vi "FaulhaberV3-Ascii_V1.vi"() -> (1 "searchnames":string[](array[string]), 2 "ID":u32[](array[numeric]), 3 "Faulhaber Objects":T3(array[cluster]))   [LabVIEW 2011] (continued)
 595132431, 595132432, 595132433, 595132434, 595132435, 595132436, 595132437, 595132438, 595132439, 595197952, 595197953, 595197954, 595197955, 595197956, 595197957, 595197958, 595197959, 595197966, 595197967, 595197968, 595197969, 595197970, 595197971, 595197972, 595197973, 595197974, 595197975, 595263488, 595263489, 595263490, 595263491, 595263492, 595263493, 595263494, 595263495, 595263502, 595263503, 595263504, 595263505, 595263506, 595263507, 595263508, 595263509, 595263510, 595263511, 595591168, 595591169, 595591170, 595591171, 595591172, 595591173, 595656704, 595656705, 595656706, 595656707, 595656708, 595656709, 595656710, 595656711, 595656712, 595722240, 595722241, 595722242, 595722243, 596574208, 596574209, 602931200, 602931201, 602931202, 602931203, 602931204, 602931205, 602931206, 602996736, 602996737, 602996738, 603127808, 603127809, 603127810, 603127811, 603127812, 603127813, 603979776, 603979777, 603979778, 603979779, 603979780, 603979781, 603979782, 603979783, 604045312, 604241920, 604307456, 604372992, 604438528, 604504064, 605028352, 605028353, 620756992, 620756993, 620756994, 620756995, 620756996, 620756997, 620756998, 620756999, 620757000, 620757001, 620757002, 620757003, 620757004, 620757005, 620757006, 620822528, 620822529, 620822530, 620822531, 620822532, 620822533, 620822534, 620822535, 620822536, 620822537, 620822538, 620822539, 620822540, 620822541, 620822542, 620888064, 620888065, 620888066, 620888067, 620888068, 620888069, 620888070, 620888071, 620888072, 620888073, 620888074, 620888075, 620888076, 620888077, 620953600, 621019136, 621019137, 621019138, 621019139, 621019140, 621019141, 621019142, 621019143, 621019144, 621019145, 621019146, 621019147, 621019148, 621150208, 621150209, 621150210, 621150211, 621150212, 621150213, 621150214, 621150215, 621150216, 621150217, 621150218, 621150219, 621150220, 621150221, 621150222, 621150223, 621150224, 621150225, 621150226, 621150227, 621150228, 621150229, 621150230, 621150231, 621150232, 621150233, 621150234, 621150235, 621150236, 621150237, 621150238, 621150239, 621150240, 621150241, 621150242, 621150243, 621150244, 621150245, 621150246, 621150247, 621150248, 621150249, 621150250, 621150251, 621150252, 621150253, 621150254, 621150255, 621150256, 621150257, 621150258, 621150259, 621150260, 621150261, 621150262, 621150263, 621150264, 621150265, 621150266, 621150267, 621150268, 621150269, 621150270, 621150271, 621150272, 621412352, 621740032, 637534208, 637534209, 637534210, 637599744, 637599745, 637599746, 637599747, 637665280, 637665281, 637665282, 637665283, 637730816, 637730817, 637730818, 637796352, 637861888, 638582784, 638582785, 638582786, 638582787, 805306368, 805306369, 805306370, 805306371, 805306372, 805306373, 805306374, 805306375, 805306376, 805371904, 805371905, 805371906, 805371907, 805371908, 805371909, 805371911, 805371912, 805371913, 805371914, 805437440, 805502976, 805568512, 805568513, 805568514, 805634048, 805634049, 805634050, 805634051, 805634052, 805634053, 805634054, 805634055, 805634056, 805634057, 805634058, 805634059, 805634060, 805634061, 805634062, 805634063, 805634064, 805634065, 805634066, 805634067, 805634068, 805634069, 805634070, 805634071, 805634072, 805634073, 805634074, 805699584, 805699585, 805699586, 805699587, 805699588, 805699589, 805699590, 805699591, 805699592, 805699593, 805699594, 805699595, 805699596, 805699597, 805699598, 805699599, 806289408, 806354944, 806354945, 806354946, 806354947, 806354948, 806354949, 806354950, 806354951, 806354952, 806354953, 806354954, 806354955, 806354956, 806354957, 806354958, 806354959, 806354960, 1611071488, 1614807040, 1614872576, 1616510976, 1616576512, 1616642048, 1616707584, 1616773120, 1616904192, 1616969728, 1617035264, 1617100800, 1617166336, 1617231872, 1617297408, 1617362944, 1617428480, 1617625088, 1617690624, 1617756160, 1617821696, 1617887232, 1617952768, 1618018304, 1618083840, 1618214912, 1618411520, 1618477056, 1618608128, 1618673664, 1618673665, 1618673666, 1618739200, 1618804736, 1618804737, 1618804738, 1618870272, 1619001344, 1619066880, 1619197952, 1619263488, 1619329024, 1619394560, 1619984384, 1619984385, 1619984386, 1620049920, 1620049921, 1620049922, 1620115456, 1620115457, 1620115458, 1620180992, 1620180993, 1620180994, 1620443136, 1620443137, 1620443138, 1620574208, 1620639744, 1620639745, 1620639746, 1620705280, 1622147072, 1622212608, 1622278144, 1622671360, 1622736896, 1622802432, 1622867968, 1622933504, 1622999040, 1623523328, 1623588864, 1624571904, 1624637440, 1624702976, 1624768512, 1625292800, 1625358336, 1626472448, 1626603520, 1627193344, 1627324416, 1677918208, 1694629888, 1694695424] format="%08x", 3 "Faulhaber Objects":T3(array[cluster])=[{"ID"=268435456, "Name"="Device type", "type"=enum."U32", "rw"=enum."ro", "lowLimit"="", "highLimit"="", "Default"="0x420192", "Kommentart"=""}, {"ID"=268500992, "Name"="Error register", "type"=enum."U8", "rw"=enum."ro", "lowLimit"="", "highLimit"="", "Default"="", "Kommentart"=""}, {"ID"=268632064, "Name"="Pre-defined error field_Number of errors", "type"=enum."U8", "rw"=enum."rw", "lowLimit"="0", "highLimit"="255", "Default"="0", "Kommentart"=""}, {"ID"=268632065, "Name"="Pre-defined error field_Standard error field 1", "type"=enum."U32", "rw"=enum."ro", "lowLimit"="", "highLimit"="", "Default"="0x0", "Kommentart"=""}, {"ID"=268632066, "Name"="Pre-defined error field_Standard error field 2", "type"=enum."U32", "rw"=enum."ro", "lowLimit"="", "highLimit"="", "Default"="0x0", "Kommentart"=""}, {"ID"=268632067, "Name"="Pre-defined error field_Standard error field 3", "type"=enum."U32", "rw"=enum."ro", "lowLimit"="", "highLimit"="", "Default"="0x0", "Kommentart"=""}, {"ID"=268632068, "Name"="Pre-defined error field_Standard error field 4", "type"=enum."U32", "rw"=enum."ro", "lowLimit"="", "highLimit"="", "Default"="0x0", "Kommentart"=""}, {"ID"=268632069, "Name"="Pre-defined error field_Standard error field 5", "type"=enum."U32", "rw"=enum."ro", "lowLimit"="", "highLimit"="", "Default"="0x0", "Kommentart"=""}, {"ID"=268632070, "Name"="Pre-defined error field_Standard error field 6", "type"=enum."U32", "rw"=enum."ro", "lowLimit"="", "highLimit"="", "Default"="0x0", "Kommentart"=""}, {"ID"=268632071, "Name"="Pre-defined error field_Standard error field 7", "type"=enum."U32", "rw"=enum."ro", "lowLimit"="", "highLimit"="", "Default"="0x0", "Kommentart"=""}, {"ID"=268632072, "Name"="Pre-defined error field_Standard error field 8", "type"=enum."U32", "rw"=enum."ro", "lowLimit"="", "highLimit"="", "Default"="0x0", "Kommentart"=""}, {"ID"=268763136, "Name"="COB-ID SYNC", "type"=enum."U32", "rw"=enum."rw", "lowLimit"="1", "highLimit"="4294967295", "Default"="0x80", "Kommentart"=""}, {"ID"=268959744, "Name"="Manufacturer device name", "type"=enum."string", "rw"=enum."const", "lowLimit"="", "highLimit"="", "Default"="", "Kommentart"=""}, {"ID"=269025280, "Name"="Manufacturer hardware version", "type"=enum."string", "rw"=enum."const", "lowLimit"="", "highLimit"="", "Default"="", "Kommentart"=""}, {"ID"=269090816, "Name"="Manufacturer software version", "type"=enum."string", "rw"=enum."const", "lowLimit"="", "highLimit"="", "Default"="", "Kommentart"=""}, {"ID"=269221888, "Name"="Guard time", "type"=enum."U16", "rw"=enum."rw", "lowLimit"="0", "highLimit"="65535", "Default"="0", "Kommentart"=""}, {"ID"=269287424, "Name"="Life time factor", "type"=enum."U8", "rw"=enum."rw", "lowLimit"="0", "highLimit"="255", "Default"="0", "Kommentart"=""}, {"ID"=269484032, "Name"="Store parameters_Number of entries", "type"=enum."U8", "rw"=enum."ro", "lowLimit"="", "highLimit"="", "Default"="9", "Kommentart"=""}, {"ID"=269484033, "Name"="Store parameters_Save all parameters", "type"=enum."U32", "rw"=enum."rw", "lowLimit"="", "highLimit"="", "Default"="", "Kommentart"=""}, {"ID"=269484034, "Name"="Store parameters_Save comm parameters", "type"=enum."U32", "rw"=enum."rw", "lowLimit"="", "highLimit"="", "Default"="", "Kommentart"=""}, {"ID"=269484035, "Name"="Store parameters_Save app parameters", "type"=enum."U32", "rw"=enum."rw", "lowLimit"="", "highLimit"="", "Default"="", "Kommentart"=""}, {"ID"=269484036, "Name"="Store parameters_Save app parameters 1", "type"=enum."U32", "rw"=enum."rw", "lowLimit"="", "highLimit"="", "Default"="", "Kommentart"=""}, {"ID"=269484037, "Name"="Store parameters_Save app parameters 2", "type"=enum."U32", "rw"=enum."rw", "lowLimit"="", "highLimit"="", "Default"="", "Kommentart"=""}, {"ID"=269484038, "Name"="Store parameters_Save cal parameters", "type"=enum."U32", "rw"=enum."ro", "lowLimit"="", "highLimit"="", "Default"="", "Kommentart"=""}, {"ID"=269484039, "Name"="Store parameters_Save factory parameter alls", "type"=enum."U32", "rw"=enum."ro", "lowLimit"="", "highLimit"="", "Default"="", "Kommentart"=""}, {"ID"=269484040, "Name"="Store parameters_Save factory parameters com", "type"=enum."U32", "rw"=enum."ro", "lowLimit"="", "highLimit"="", "Default"="", "Kommentart"=""}, {"ID"=269484041, "Name"="Store parameters_Save factory parameters app", "type"=enum."U32", "rw"=enum."ro", "lowLimit"="", "highLimit"="", "Default"="", "Kommentart"=""}, {"ID"=269549568, "Name"="Restore default parameters_Number of entries", "type"=enum."U8", "rw"=enum."ro", "lowLimit"="", "highLimit"="", "Default"="6", "Kommentart"=""}, {"ID"=269549569, "Name"="Restore default parameters_Restore all default parameters", "type"=enum."U32", "rw"=enum."rw", "lowLimit"="", "highLimit"="", "Default"="", "Kommentart"=""}, {"ID"=269549570, "Name"="Restore default parameters_Restore comm default parameters", "type"=enum."U32", "rw"=enum."rw", "lowLimit"="", "highLimit"="", "Default"="", "Kommentart"=""}, {"ID"=269549571, "Name"="Restore default parameters_Restore app default parameters", "type"=enum."U32", "rw"=enum."rw", "lowLimit"="", "highLimit"="", "Default"="", "Kommentart"=""}, {"ID"=269549572, "Name"="Restore default parameters_Restore app saved", "type"=enum."U32", "rw"=enum."rw", "lowLimit"="", "highLimit"="", "Default"="", "Kommentart"=""}, {"ID"=269549573, "Name"="Restore default parameters_Restore app 1 saved", "type"=enum."U32", "rw"=enum."rw", "lowLimit"="", "highLimit"="", "Default"="", "Kommentart"=""}, {"ID"=269549574, "Name"="Restore default parameters_Restore app 2 saved", "type"=enum."U32", "rw"=enum."rw", "lowLimit"="", "highLimit"="", "Default"="", "Kommentart"=""}, {"ID"=269746176, "Name"="COB-ID EMCY", "type"=enum."U32", "rw"=enum."rw", "lowLimit"="", "highLimit"="", "Default"="$NODEID+0x80", "Kommentart"=""}, {"ID"=269877248, "Name"="Consumer heartbeat time_Number of entries", "type"=enum."U8", "rw"=enum."ro", "lowLimit"="", "highLimit"="", "Default"="1", "Kommentart"=""}, {"ID"=269877249, "Name"="Consumer heartbeat time_Consumer heartbeat time", "type"=enum."U32", "rw"=enum."rw", "lowLimit"="0", "highLimit"="0x007FFFFF", "Default"="0x0", "Kommentart"=""}, {"ID"=269942784, "Name"="Producer heartbeat time", "type"=enum."U16", "rw"=enum."rw", "lowLimit"="0", "highLimit"="65535", "Default"="0", "Kommentart"=""}, {"ID"=270008320, "Name"="Identity object_Number of entries", "type"=enum."U8", "rw"=enum."ro", "lowLimit"="", "highLimit"="", "Default"="4", "Kommentart"=""}, {"ID"=270008321, "Name"="Identity object_Vendor ID", "type"=enum."U32", "rw"=enum."ro", "lowLimit"="", "highLimit"="", "Default"="327", "Kommentart"=""}, {"ID"=270008322, "Name"="Identity object_Product code", "type"=enum."U32", "rw"=enum."ro", "lowLimit"="", "highLimit"="", "Default"="", "Kommentart"=""}, {"ID"=270008323, "Name"="Identity object_Revision number", "type"=enum."U32", "rw"=enum."ro", "lowLimit"="0x0", "highLimit"="", "Default"="", "Kommentart"=""}, {"ID"=270008324, "Name"="Identity object_Serial number", "type"=enum."U32", "rw"=enum."ro", "lowLimit"="", "highLimit"="", "Default"="", "Kommentart"=""}, {"ID"=271122432, "Name"="Error behaviour / Number of error classes_Number of error classes", "type"=enum."U8", "rw"=enum."ro", "lowLimit"="", "highLimit"="", "Default"="1", "Kommentart"=""}, {"ID"=271122433, "Name"="Error behaviour / Number of error classes_Communication error", "type"=enum."U8", "rw"=enum."unknown", "lowLimit"="", "highLimit"="", "Default"="", "Kommentart"=""}, {"ID"=301989888, "Name"="Server SDO parameter_Number of entries", "type"=enum."U8", "rw"=enum."ro", "lowLimit"="", "highLimit"="", "Default"="2", "Kommentart"=""}, {"ID"=301989889, "Name"="Server SDO parameter_COB-ID client to server (rx)", "type"=enum."U32", "rw"=enum."ro", "lowLimit"="", "highLimit"="", "Default"="$NODEID+0x600", "Kommentart"=""}, {"ID"=301989890, "Name"="Server SDO parameter_COB-ID server to client (tx)", "type"=enum."U32", "rw"=enum."ro", "lowLimit"="", "highLimit"="", "Default"="$NODEID+0x580", "Kommentart"=""}, {"ID"=335544320, "Name"="Receive PDO1 parameter_Number of entries", "type"=enum."U8", "rw"=enum."ro", "lowLimit"="", "highLimit"="", "Default"="2", "Kommentart"=""}, {"ID"=335544321, "Name"="Receive PDO1 parameter_COB-ID used by RxPDO1", "type"=enum."U32", "rw"=enum."rw", "lowLimit"="1", "highLimit"="4294967295", "Default"="$NODEID+0x200", "Kommentart"=""}, {"ID"=335544322, "Name"="Receive PDO1 parameter_Transmission type", "type"=enum."U8", "rw"=enum."rw", "lowLimit"="0", "highLimit"="255", "Default"="255", "Kommentart"=""}, {"ID"=335609856, "Name"="Receive PDO2 parameter_Number of entries", "type"=enum."U8", "rw"=enum."ro", "lowLimit"="", "highLimit"="", "Default"="2", "Kommentart"=""}, {"ID"=335609857, "Name"="Receive PDO2 parameter_COB-ID used by RxPDO2", "type"=enum."U32", "rw"=enum."rw", "lowLimit"="1", "highLimit"="4294967295", "Default"="$NODEID+0x300", "Kommentart"=""}, {"ID"=335609858, "Name"="Receive PDO2 parameter_Transmission type", "type"=enum."U8", "rw"=enum."rw", "lowLimit"="0", "highLimit"="255", "Default"="255", "Kommentart"=""}, {"ID"=335675392, "Name"="Receive PDO3 parameters_Number of entries", "type"=enum."U8", "rw"=enum."ro", "lowLimit"="", "highLimit"="", "Default"="2", "Kommentart"=""}, {"ID"=335675393, "Name"="Receive PDO3 parameters_COB-ID used by RxPDO3", "type"=enum."U32", "rw"=enum."rw", "lowLimit"="1", "highLimit"="4294967295", "Default"="$NODEID+0x400", "Kommentart"=""}, {"ID"=335675394, "Name"="Receive PDO3 parameters_Transmission type", "type"=enum."U8", "rw"=enum."rw", "lowLimit"="0", "highLimit"="255", "Default"="255", "Kommentart"=""}, {"ID"=335740928, "Name"="Receive PDO4 parameter_Number of entries", "type"=enum."U8", "rw"=enum."ro", "lowLimit"="", "highLimit"="", "Default"="2", "Kommentart"=""}, {"ID"=335740929, "Name"="Receive PDO4 parameter_COB-ID used by RxPDO4", "type"=enum."U32", "rw"=enum."rw", "lowLimit"="1", "highLimit"="4294967295", "Default"="$NODEID+0x500", "Kommentart"=""}, {"ID"=335740930, "Name"="Receive PDO4 parameter_Transmission type", "type"=enum."U8", "rw"=enum."rw", "lowLimit"="0", "highLimit"="255", "Default"="255", "Kommentart"=""}, {"ID"=369098752, "Name"="Receive PDO1 mapping / Number of mapped objects_Number of mapped objects", "type"=enum."U8", "rw"=enum."rw", "lowLimit"="0", "highLimit"="4", "Default"="1", "Kommentart"=""}, {"ID"=369098753, "Name"="Receive PDO1 mapping / Number of mapped objects_RxPDO 1 mapping entry 1", "type"=enum."U32", "rw"=enum."rw", "lowLimit"="0", "highLimit"="4294967295", "Default"="0x60400010", "Kommentart"=""}, {"ID"=369098754, "Name"="Receive PDO1 mapping / Number of mapped objects_RxPDO 1 Mapping entry 2", "type"=enum."U32", "rw"=enum."rw", "lowLimit"="0", "highLimit"="4294967295", "Default"="0x0", "Kommentart"=""}, {"ID"=369098755, "Name"="Receive PDO1 mapping / Number of mapped objects_RxPDO 1 Mapping entry 3", "type"=enum."U32", "rw"=enum."rw", "lowLimit"="0", "highLimit"="4294967295", "Default"="0x0", "Kommentart"=""}, {"ID"=369098756, "Name"="Receive PDO1 mapping / Number of mapped objects_RxPDO 1 Mapping entry 4", "type"=enum."U32", "rw"=enum."rw", "lowLimit"="0", "highLimit"="4294967295", "Default"="0x0", "Kommentart"=""}, {"ID"=369164288, "Name"="Receive PDO2 mapping / Number of mapped objects_Number of mapped objects", "type"=enum."U8", "rw"=enum."rw", "lowLimit"="0", "highLimit"="4", "Default"="2", "Kommentart"=""}, {"ID"=369164289, "Name"="Receive PDO2 mapping / Number of mapped objects_RxPDO2 mapping entry 1", "type"=enum."U32", "rw"=enum."rw", "lowLimit"="0", "highLimit"="4294967295", "Default"="0x60400010", "Kommentart"=""}, {"ID"=369164290, "Name"="Receive PDO2 mapping / Number of mapped objects_RxPDO2 mapping entry 2", "type"=enum."U32", "rw"=enum."rw", "lowLimit"="0", "highLimit"="4294967295", "Default"="0x607A0020", "Kommentart"=""}, {"ID"=369164291, "Name"="Receive PDO2 mapping / Number of mapped objects_RxPDO2 mapping entry 3", "type"=enum."U32", "rw"=enum."rw", "lowLimit"="0", "highLimit"="4294967295", "Default"="0x0", "Kommentart"=""}, {"ID"=369164292, "Name"="Receive PDO2 mapping / Number of mapped objects_RxPDO2 mapping entry 4", "type"=enum."U32", "rw"=enum."rw", "lowLimit"="0", "highLimit"="4294967295", "Default"="0x0", "Kommentart"=""}, {"ID"=369229824, "Name"="Receive PDO3 mapping / Number of mapped objects_Number of mapped objects", "type"=enum."U8", "rw"=enum."rw", "lowLimit"="0", "highLimit"="4", "Default"="2", "Kommentart"=""}, {"ID"=369229825, "Name"="Receive PDO3 mapping / Number of mapped objects_RxPDO3 mapping entry 1", "type"=enum."U32", "rw"=enum."rw", "lowLimit"="0", "highLimit"="4294967295", "Default"="0x60400010", "Kommentart"=""}, {"ID"=369229826, "Name"="Receive PDO3 mapping / Number of mapped objects_RxPDO3 mapping entry 2", "type"=enum."U32", "rw"=enum."rw", "lowLimit"="0", "highLimit"="4294967295", "Default"="0x60FF0020", "Kommentart"=""}, {"ID"=369229827, "Name"="Receive PDO3 mapping / Number of mapped objects_RxPDO3 mapping entry 3", "type"=enum."U32", "rw"=enum."rw", "lowLimit"="0", "highLimit"="4294967295", "Default"="0x0", "Kommentart"=""}, {"ID"=369229828, "Name"="Receive PDO3 mapping / Number of mapped objects_RxPDO3 mapping entry 4", "type"=enum."U32", "rw"=enum."rw", "lowLimit"="0", "highLimit"="4294967295", "Default"="0x0", "Kommentart"=""}, {"ID"=369295360, "Name"="Receive PDO4 mapping / Number of mapped objects_Number of mapped objects", "type"=enum."U8", "rw"=enum."rw", "lowLimit"="0", "highLimit"="4", "Default"="2", "Kommentart"=""}, {"ID"=369295361, "Name"="Receive PDO4 mapping / Number of mapped objects_RxPDO4 mapping entry 1", "type"=enum."U32", "rw"=enum."rw", "lowLimit"="0", "highLimit"="4294967295", "Default"="0x60400010", "Kommentart"=""}, {"ID"=369295362, "Name"="Receive PDO4 mapping / Number of mapped objects_RxPDO4 mapping entry 2", "type"=enum."U32", "rw"=enum."rw", "lowLimit"="0", "highLimit"="4294967295", "Default"="0x60710010", "Kommentart"=""}, {"ID"=369295363, "Name"="Receive PDO4 mapping / Number of mapped objects_RxPDO4 mapping entry 3", "type"=enum."U32", "rw"=enum."rw", "lowLimit"="0", "highLimit"="4294967295", "Default"="0x0", "Kommentart"=""}, {"ID"=369295364, "Name"="Receive PDO4 mapping / Number of mapped objects_RxPDO4 mapping entry 4", "type"=enum."U32", "rw"=enum."rw", "lowLimit"="0", "highLimit"="4294967295", "Default"="0x0", "Kommentart"=""}, {"ID"=402653184, "Name"="Transmit PDO1 parameter_Number of entries", "type"=enum."U8", "rw"=enum."ro", "lowLimit"="", "highLimit"="", "Default"="5", "Kommentart"=""}, {"ID"=402653185, "Name"="Transmit PDO1 parameter_COB-ID used by TxPDO1", "type"=enum."U32", "rw"=enum."rw", "lowLimit"="1", "highLimit"="4294967295", "Default"="$NODEID+0x180", "Kommentart"=""}, {"ID"=402653186, "Name"="Transmit PDO1 parameter_Transmission type", "type"=enum."U8", "rw"=enum."rw", "lowLimit"="0", "highLimit"="255", "Default"="255", "Kommentart"=""}, {"ID"=402653189, "Name"="Transmit PDO1 parameter_Eventtimer", "type"=enum."U16", "rw"=enum."rw", "lowLimit"="0", "highLimit"="65535", "Default"="0", "Kommentart"=""}, {"ID"=402718720, "Name"="Transmit PDO2 parameter_Number of entries", "type"=enum."U8", "rw"=enum."ro", "lowLimit"="", "highLimit"="", "Default"="5", "Kommentart"=""}, {"ID"=402718721, "Name"="Transmit PDO2 parameter_COB-ID used by TxPDO2", "type"=enum."U32", "rw"=enum."rw", "lowLimit"="1", "highLimit"="4294967295", "Default"="$NODEID+0x280", "Kommentart"=""}, {"ID"=402718722, "Name"="Transmit PDO2 parameter_Transmission type", "type"=enum."U8", "rw"=enum."rw", "lowLimit"="0", "highLimit"="255", "Default"="255", "Kommentart"=""}, {"ID"=402718725, "Name"="Transmit PDO2 parameter_Eventtimer", "type"=enum."U16", "rw"=enum."rw", "lowLimit"="0", "highLimit"="65535", "Default"="0", "Kommentart"=""}, {"ID"=402784256, "Name"="Transmit PDO3 parameter_Number of entries", "type"=enum."U8", "rw"=enum."ro", "lowLimit"="", "highLimit"="", "Default"="5", "Kommentart"=""}, {"ID"=402784257, "Name"="Transmit PDO3 parameter_COB-ID used by TxPDO3", "type"=enum."U32", "rw"=enum."rw", "lowLimit"="1", "highLimit"="4294967295", "Default"="$NODEID+0x380", "Kommentart"=""}, {"ID"=402784258, "Name"="Transmit PDO3 parameter_Transmission type", "type"=enum."U8", "rw"=enum."rw", "lowLimit"="0", "highLimit"="255", "Default"="255", "Kommentart"=""}, {"ID"=402784261, "Name"="Transmit PDO3 parameter_Eventtimer", "type"=enum."U16", "rw"=enum."rw", "lowLimit"="0", "highLimit"="65535", "Default"="0", "Kommentart"=""}, {"ID"=402849792, "Name"="Transmit PDO4 parameter_Number of entries", "type"=enum."U8", "rw"=enum."ro", "lowLimit"="", "highLimit"="", "Default"="5", "Kommentart"=""}, {"ID"=402849793, "Name"="Transmit PDO4 parameter_COB-ID used by TxPDO4", "type"=enum."U32", "rw"=enum."rw", "lowLimit"="1", "highLimit"="4294967295", "Default"="$NODEID+0x480", "Kommentart"=""}, {"ID"=402849794, "Name"="Transmit PDO4 parameter_Transmission type", "type"=enum."U8", "rw"=enum."rw", "lowLimit"="0", "highLimit"="255", "Default"="255", "Kommentart"=""}, {"ID"=402849797, "Name"="Transmit PDO4 parameter_Eventtimer", "type"=enum."U16", "rw"=enum."rw", "lowLimit"="0", "highLimit"="65535", "Default"="0", "Kommentart"=""}, {"ID"=436207616, "Name"="Transmit PDO1 mapping  / Number of mapped objects_Number of mapped objects", "type"=enum."U8", "rw"=enum."rw", "lowLimit"="0", "highLimit"="4", "Default"="1", "Kommentart"=""}, {"ID"=436207617, "Name"="Transmit PDO1 mapping  / Number of mapped objects_TPDO1 mapping entry 1", "type"=enum."U32", "rw"=enum."rw", "lowLimit"="0", "highLimit"="4294967295", "Default"="0x60410010", "Kommentart"=""}, {"ID"=436207618, "Name"="Transmit PDO1 mapping  / Number of mapped objects_TPDO1 mapping entry 2", "type"=enum."U32", "rw"=enum."rw", "lowLimit"="0", "highLimit"="4294967295", "Default"="0x0", "Kommentart"=""}, {"ID"=436207619, "Name"="Transmit PDO1 mapping  / Number of mapped objects_TxPDO1 mapping entry 3", "type"=enum."U32", "rw"=enum."rw", "lowLimit"="0", "highLimit"="4294967295", "Default"="0x0", "Kommentart"=""}, {"ID"=436207620, "Name"="Transmit PDO1 mapping  / Number of mapped objects_TxPDO1 mapping entry 4", "type"=enum."U32", "rw"=enum."rw", "lowLimit"="0", "highLimit"="4294967295", "Default"="0x0", "Kommentart"=""}, {"ID"=436273152, "Name"="Transmit PDO2 mapping  / Number of mapped objects_Number of mapped objects", "type"=enum."U8", "rw"=enum."rw", "lowLimit"="0", "highLimit"="4", "Default"="2", "Kommentart"=""}, {"ID"=436273153, "Name"="Transmit PDO2 mapping  / Number of mapped objects_TxPDO1 mapping entry 1", "type"=enum."U32", "rw"=enum."rw", "lowLimit"="0", "highLimit"="4294967295", "Default"="0x60410010", "Kommentart"=""}, {"ID"=436273154, "Name"="Transmit PDO2 mapping  / Number of mapped objects_TxPDO2 mapping entry 2", "type"=enum."U32", "rw"=enum."rw", "lowLimit"="0", "highLimit"="4294967295", "Default"="0x60640020", "Kommentart"=""}, {"ID"=436273155, "Name"="Transmit PDO2 mapping  / Number of mapped objects_TxPDO3 mapping entry 3", "type"=enum."U32", "rw"=enum."rw", "lowLimit"="0", "highLimit"="4294967295", "Default"="0x0", "Kommentart"=""}, {"ID"=436273156, "Name"="Transmit PDO2 mapping  / Number of mapped objects_TxPDO4 mapping entry 4", "type"=enum."U32", "rw"=enum."rw", "lowLimit"="0", "highLimit"="4294967295", "Default"="0x0", "Kommentart"=""}, {"ID"=436338688, "Name"="Transmit PDO3 mapping  / Number of mapped objects_Number of mapped objects", "type"=enum."U8", "rw"=enum."rw", "lowLimit"="0", "highLimit"="4", "Default"="2", "Kommentart"=""}, {"ID"=436338689, "Name"="Transmit PDO3 mapping  / Number of mapped objects_TxPDO3 mapping entry 1", "type"=enum."U32", "rw"=enum."rw", "lowLimit"="0", "highLimit"="4294967295", "Default"="0x60410010", "Kommentart"=""}, {"ID"=436338690, "Name"="Transmit PDO3 mapping  / Number of mapped objects_TxPDO3 mapping entry 2", "type"=enum."U32", "rw"=enum."rw", "lowLimit"="0", "highLimit"="4294967295", "Default"="0x606C0020", "Kommentart"=""}, {"ID"=436338691, "Name"="Transmit PDO3 mapping  / Number of mapped objects_TxPDO3 mapping entry 3", "type"=enum."U32", "rw"=enum."rw", "lowLimit"="0", "highLimit"="4294967295", "Default"="0x0", "Kommentart"=""}, {"ID"=436338692, "Name"="Transmit PDO3 mapping  / Number of mapped objects_TxPDO3 mapping entry 4", "type"=enum."U32", "rw"=enum."rw", "lowLimit"="0", "highLimit"="4294967295", "Default"="0x0", "Kommentart"=""}, {"ID"=436404224, "Name"="Transmit PDO4 mapping  / Number of mapped objects_Number of mapped objects", "type"=enum."U8", "rw"=enum."rw", "lowLimit"="0", "highLimit"="4", "Default"="2", "Kommentart"=""}, {"ID"=436404225, "Name"="Transmit PDO4 mapping  / Number of mapped objects_TxPDO4 mapping entry 1", "type"=enum."U32", "rw"=enum."rw", "lowLimit"="0", "highLimit"="4294967295", "Default"="0x60410010", "Kommentart"=""}, {"ID"=436404226, "Name"="Transmit PDO4 mapping  / Number of mapped objects_TxPDO4 mapping entry 2", "type"=enum."U32", "rw"=enum."rw", "lowLimit"="0", "highLimit"="4294967295", "Default"="0x60770010", "Kommentart"=""}, {"ID"=436404227, "Name"="Transmit PDO4 mapping  / Number of mapped objects_TxPDO4 mapping entry 3", "type"=enum."U32", "rw"=enum."rw", "lowLimit"="0", "highLimit"="4294967295", "Default"="0x0", "Kommentart"=""}, {"ID"=436404228, "Name"="Transmit PDO4 mapping  / Number of mapped objects_TxPDO4 mapping entry 4", "type"=enum."U32", "rw"=enum."rw", "lowLimit"="0", "highLimit"="4294967295", "Default"="0x0", "Kommentart"=""}, {"ID"=587202560, "Name"="Number of I/Os_Number of entries", "type"=enum."U8", "rw"=enum."ro", "lowLimit"="", "highLimit"="", "Default"="4", "Kommentart"=""}, {"ID"=587202561, "Name"="Number of I/Os_Number of digital inputs", "type"=enum."U8", "rw"=enum."ro", "lowLimit"="", "highLimit"="", "Default"="", "Kommentart"=""}, {"ID"=587202562, "Name"="Number of I/Os_Number of digital outputs", "type"=enum."U8", "rw"=enum."ro", "lowLimit"="", "highLimit"="", "Default"="", "Kommentart"=""}, {"ID"=587202563, "Name"="Number of I/Os_Number of analog inputs", "type"=enum."U8", "rw"=enum."ro", "lowLimit"="", "highLimit"="", "Default"="", "Kommentart"=""}, {"ID"=587202564, "Name"="Number of I/Os_Number of emulated digital inputs", "type"=enum."U8", "rw"=enum."unknown", "lowLimit"="", "highLimit"="", "Default"="", "Kommentart"=""}, {"ID"=588251136, "Name"="Digital input settings_Number of entries", "type"=enum."U8", "rw"=enum."ro", "lowLimit"="", "highLimit"="", "Default"="18", "Kommentart"=""}, {"ID"=588251137, "Name"="Digital input settings_Select lower limit switch inputs", "type"=enum."U8", "rw"=enum."unknown", "lowLimit"="", "highLimit"="", "Default"="", "Kommentart"=""}, {"ID"=588251138, "Name"="Digital input settings_Select upper limit switch inputs", "type"=enum."U8", "rw"=enum."unknown", "lowLimit"="", "highLimit"="", "Default"="", "Kommentart"=""}, {"ID"=588251139, "Name"="Digital input settings_Limit switch option code", "type"=enum."S16", "rw"=enum."unknown", "lowLimit"="", "highLimit"="", "Default"="", "Kommentart"=""}, {"ID"=588251140, "Name"="Digital input settings_Select reference switch input", "type"=enum."U8", "rw"=enum."rw", "lowLimit"="0", "highLimit"="8", "Default"="0", "Kommentart"=""}, {"ID"=588251141, "Name"="Digital input settings_Emulated input threshold level", "type"=enum."U8", "rw"=enum."rw", "lowLimit"="0", "highLimit"="0x03", "Default"="0x00", "Kommentart"=""}, {"ID"=588251142, "Name"="Digital input settings_Select stop input", "type"=enum."U8", "rw"=enum."unknown", "lowLimit"="", "highLimit"="", "Default"="", "Kommentart"=""}, {"ID"=588251144, "Name"="Digital input settings_Debug Write Digital Input Values", "type"=enum."U8", "rw"=enum."wo", "lowLimit"="0", "highLimit"="255", "Default"="", "Kommentart"=""}, {"ID"=588251145, "Name"="Digital input settings_Debug Write Brake / Fault Pin", "type"=enum."U8", "rw"=enum."wo", "lowLimit"="0", "highLimit"="255", "Default"="", "Kommentart"=""}, {"ID"=588251151, "Name"="Digital input settings_Select digital inputs used", "type"=enum."U8", "rw"=enum."rw", "lowLimit"="0", "highLimit"="255", "Default"="0xFF", "Kommentart"=""}, {"ID"=588251152, "Name"="Digital input settings_Input polarity", "type"=enum."U8", "rw"=enum."rw", "lowLimit"="0", "highLimit"="255", "Default"="0x0", "Kommentart"=""}, {"ID"=588251153, "Name"="Digital input settings_Input threshold level", "type"=enum."U8", "rw"=enum."unknown", "lowLimit"="", "highLimit"="", "Default"="", "Kommentart"=""}, {"ID"=588251154, "Name"="Digital input settings_Input filter active", "type"=enum."U8", "rw"=enum."rw", "lowLimit"="0", "highLimit"="255", "Default"="0x0", "Kommentart"=""}, {"ID"=588316672, "Name"="Digital I/O status_Number of entries", "type"=enum."U8", "rw"=enum."ro", "lowLimit"="", "highLimit"="", "Default"="4", "Kommentart"=""}, {"ID"=588316673, "Name"="Digital I/O status_Digital input logical state", "type"=enum."U8", "rw"=enum."ro", "lowLimit"="0x0", "highLimit"="", "Default"="", "Kommentart"=""}, {"ID"=588316674, "Name"="Digital I/O status_Digital input physical state", "type"=enum."U8", "rw"=enum."ro", "lowLimit"="0x0", "highLimit"="", "Default"="", "Kommentart"=""}, {"ID"=588316675, "Name"="Digital I/O status_Digital output status", "type"=enum."U8", "rw"=enum."ro", "lowLimit"="0x0", "highLimit"="", "Default"="", "Kommentart"=""}, {"ID"=588316676, "Name"="Digital I/O status_Write digital outputs", "type"=enum."U16", "rw"=enum."rw", "lowLimit"="0", "highLimit"="65535", "Default"="0x0", "Kommentart"=""}, {"ID"=588382208, "Name"="Digital output settings_Number of entries", "type"=enum."U8", "rw"=enum."ro", "lowLimit"="", "highLimit"="", "Default"="16", "Kommentart"=""}, {"ID"=588382209, "Name"="Digital output settings_Select fault output pin", "type"=enum."U8", "rw"=enum."rw", "lowLimit"="0", "highLimit"="255", "Default"="0", "Kommentart"=""}, {"ID"=588382210, "Name"="Digital output settings_Select brake control pin", "type"=enum."U8", "rw"=enum."rw", "lowLimit"="0", "highLimit"="255", "Default"="0", "Kommentart"=""}, {"ID"=588382211, "Name"="Digital output settings_Brake delay time", "type"=enum."U8", "rw"=enum."rw", "lowLimit"="0", "highLimit"="255", "Default"="0", "Kommentart"=""}, {"ID"=588382216, "Name"="Digital output settings_DiagOut 1 pin selection", "type"=enum."U8", "rw"=enum."rw", "lowLimit"="0", "highLimit"="255", "Default"="0", "Kommentart"=""}, {"ID"=588382217, "Name"="Digital output settings_DiagOut 1 mask", "type"=enum."U32", "rw"=enum."rw", "lowLimit"="0", "highLimit"="4294967295", "Default"="0x0", "Kommentart"=""}, {"ID"=588382218, "Name"="Digital output settings_DiagOut 2 pin selection", "type"=enum."U8", "rw"=enum."rw", "lowLimit"="0", "highLimit"="255", "Default"="0", "Kommentart"=""}, {"ID"=588382219, "Name"="Digital output settings_DiagOut 2 mask", "type"=enum."U32", "rw"=enum."rw", "lowLimit"="0", "highLimit"="4294967295", "Default"="0x0", "Kommentart"=""}, {"ID"=588382220, "Name"="Digital output settings_DiagOut 3 pin selection", "type"=enum."U8", "rw"=enum."rw", "lowLimit"="0", "highLimit"="255", "Default"="0", "Kommentart"=""}, {"ID"=588382221, "Name"="Digital output settings_DiagOut 3 mask", "type"=enum."U32", "rw"=enum."rw", "lowLimit"="0", "highLimit"="4294967295", "Default"="0x0", "Kommentart"=""}, {"ID"=588382222, "Name"="Digital output settings_DiagOut 4 pin selection", "type"=enum."U8", "rw"=enum."rw", "lowLimit"="0", "highLimit"="255", "Default"="0", "Kommentart"=""}, {"ID"=588382223, "Name"="Digital output settings_DiagOut 4 mask", "type"=enum."U32", "rw"=enum."rw", "lowLimit"="0", "highLimit"="4294967295", "Default"="0x0", "Kommentart"=""}, {"ID"=588382224, "Name"="Digital output settings_Output polarity", "type"=enum."U8", "rw"=enum."rw", "lowLimit"="0", "highLimit"="0x07", "Default"="0x0", "Kommentart"=""}, {"ID"=588447744, "Name"="Analog inputs_Number of entries", "type"=enum."U8", "rw"=enum."ro", "lowLimit"="", "highLimit"="", "Default"="26", "Kommentart"=""}, {"ID"=588447745, "Name"="Analog inputs_AnIn 1 gain (numerator/divisor)", "type"=enum."S32", "rw"=enum."rw", "lowLimit"="-2147483648", "highLimit"="2147483647", "Default"="0x7FFF8000", "Kommentart"=""}, {"ID"=588447746, "Name"="Analog inputs_AnIn 1 offset", "type"=enum."S16", "rw"=enum."rw", "lowLimit"="-32768", "highLimit"="32767", "Default"="0", "Kommentart"=""}, {"ID"=588447747, "Name"="Analog inputs_AnIn 1 filter time", "type"=enum."U16", "rw"=enum."rw", "lowLimit"="0", "highLimit"="65535", "Default"="0", "Kommentart"=""}, {"ID"=588447748, "Name"="Analog inputs_AnIn 1 user scaled value", "type"=enum."S32", "rw"=enum."ro", "lowLimit"="", "highLimit"="", "Default"="", "Kommentart"=""}, {"ID"=588447749, "Name"="Analog inputs_AnIn 1 resolution as encoder", "type"=enum."U16", "rw"=enum."rw", "lowLimit"="0", "highLimit"="65535", "Default"="1000", "Kommentart"=""}, {"ID"=588447750, "Name"="Analog inputs_AnIn 1 min input limit", "type"=enum."S16", "rw"=enum."rw", "lowLimit"="-32768", "highLimit"="32767", "Default"="-32768", "Kommentart"=""}, {"ID"=588447751, "Name"="Analog inputs_AnIn 1 max input limit", "type"=enum."S16", "rw"=enum."rw", "lowLimit"="-32768", "highLimit"="32767", "Default"="32767", "Kommentart"=""}, {"ID"=588447752, "Name"="Analog inputs_AnIn 1 select dir pin", "type"=enum."U8", "rw"=enum."rw", "lowLimit"="0", "highLimit"="8", "Default"="0", "Kommentart"=""}, {"ID"=588447753, "Name"="Analog inputs_AnIn 1 virtual input value", "type"=enum."S16", "rw"=enum."rw", "lowLimit"="-32768", "highLimit"="32767", "Default"="0", "Kommentart"=""}, {"ID"=588447754, "Name"="Analog inputs_AnIn 1 enable virtual input", "type"=enum."U8", "rw"=enum."unknown", "lowLimit"="", "highLimit"="", "Default"="", "Kommentart"=""}, {"ID"=588447761, "Name"="Analog inputs_AnIn 2 gain (numerator/divisor)", "type"=enum."S32", "rw"=enum."rw", "lowLimit"="-2147483648", "highLimit"="2147483647", "Default"="0x7FFF8000", "Kommentart"=""}, {"ID"=588447762, "Name"="Analog inputs_AnIn 2 offset", "type"=enum."S16", "rw"=enum."rw", "lowLimit"="-32768", "highLimit"="32767", "Default"="0", "Kommentart"=""}, {"ID"=588447763, "Name"="Analog inputs_AnIn 2 filter time", "type"=enum."U16", "rw"=enum."rw", "lowLimit"="0", "highLimit"="65535", "Default"="0", "Kommentart"=""}, {"ID"=588447764, "Name"="Analog inputs_AnIn 2 user scaled value", "type"=enum."S32", "rw"=enum."ro", "lowLimit"="", "highLimit"="", "Default"="", "Kommentart"=""}, {"ID"=588447765, "Name"="Analog inputs_AnIn 2 resolution as encoder", "type"=enum."U16", "rw"=enum."rw", "lowLimit"="0", "highLimit"="65535", "Default"="1000", "Kommentart"=""}, {"ID"=588447766, "Name"="Analog inputs_AnIn 2 min input limit", "type"=enum."S16", "rw"=enum."rw", "lowLimit"="-32768", "highLimit"="32767", "Default"="-32768", "Kommentart"=""}, {"ID"=588447767, "Name"="Analog inputs_AnIn 2 max input limit", "type"=enum."S16", "rw"=enum."rw", "lowLimit"="-32768", "highLimit"="32767", "Default"="32767", "Kommentart"=""}, {"ID"=588447768, "Name"="Analog inputs_AnIn 2 select dir pin", "type"=enum."U8", "rw"=enum."rw", "lowLimit"="0", "highLimit"="8", "Default"="0", "Kommentart"=""}, {"ID"=588447769, "Name"="Analog inputs_AnIn 2 virtual input value", "type"=enum."S16", "rw"=enum."rw", "lowLimit"="-32768", "highLimit"="32767", "Default"="0", "Kommentart"=""}, {"ID"=588447770, "Name"="Analog inputs_AnIn 2 enable virtual input", "type"=enum."U8", "rw"=enum."unknown", "lowLimit"="", "highLimit"="", "Default"="", "Kommentart"=""}, {"ID"=588513280, "Name"="Manufacturer scaled analog input values_Number of entries", "type"=enum."U8", "rw"=enum."ro", "lowLimit"="", "highLimit"="", "Default"="12", "Kommentart"=""}, {"ID"=588513281, "Name"="Manufacturer scaled analog input values_AnIn 1 scaled value (IA)", "type"=enum."S16", "rw"=enum."ro", "lowLimit"="", "highLimit"="", "Default"="", "Kommentart"=""}, {"ID"=588513282, "Name"="Manufacturer scaled analog input values_AnIn 2 scaled value (IB)", "type"=enum."S16", "rw"=enum."ro", "lowLimit"="", "highLimit"="", "Default"="", "Kommentart"=""}, {"ID"=588513283, "Name"="Manufacturer scaled analog input values_AnIn 3 scaled value (IC)", "type"=enum."S16", "rw"=enum."ro", "lowLimit"="", "highLimit"="", "Default"="", "Kommentart"=""}, {"ID"=588513284, "Name"="Manufacturer scaled analog input values_AnIn 4 scaled value (Hall A)", "type"=enum."S16", "rw"=enum."ro", "lowLimit"="", "highLimit"="", "Default"="", "Kommentart"=""}, {"ID"=588513285, "Name"="Manufacturer scaled analog input values_AnIn 5 scaled value (Hall B)", "type"=enum."S16", "rw"=enum."ro", "lowLimit"="", "highLimit"="", "Default"="", "Kommentart"=""}, {"ID"=588513286, "Name"="Manufacturer scaled analog input values_AnIn 6 scaled value (Hall C)", "type"=enum."S16", "rw"=enum."ro", "lowLimit"="", "highLimit"="", "Default"="", "Kommentart"=""}, {"ID"=588513287, "Name"="Manufacturer scaled analog input values_AnIn 7 scaled value ", "type"=enum."S16", "rw"=enum."ro", "lowLimit"="", "highLimit"="", "Default"="", "Kommentart"=""}, {"ID"=588513288, "Name"="Manufacturer scaled analog input values_AnIn 8 scaled value ", "type"=enum."S16", "rw"=enum."ro", "lowLimit"="", "highLimit"="", "Default"="", "Kommentart"=""}, {"ID"=588513289, "Name"="Manufacturer scaled analog input values_AnIn 9 scaled value ", "type"=enum."S16", "rw"=enum."ro", "lowLimit"="", "highLimit"="", "Default"="", "Kommentart"=""}, {"ID"=588513290, "Name"="Manufacturer scaled analog input values_AnIn 10 scaled value ", "type"=enum."S16", "rw"=enum."ro", "lowLimit"="", "highLimit"="", "Default"="", "Kommentart"=""}, {"ID"=588513291, "Name"="Manufacturer scaled analog input values_AnIn 11 scaled value ", "type"=enum."S16", "rw"=enum."ro", "lowLimit"="", "highLimit"="", "Default"="", "Kommentart"=""}, {"ID"=588513292, "Name"="Manufacturer scaled analog input values_AnIn 12 scaled value ", "type"=enum."S16", "rw"=enum."ro", "lowLimit"="", "highLimit"="", "Default"="", "Kommentart"=""}, {"ID"=588578816, "Name"="Motor encoder_Number of entries", "type"=enum."U8", "rw"=enum."ro", "lowLimit"="", "highLimit"="", "Default"="10", "Kommentart"=""}, {"ID"=588578817, "Name"="Motor encoder_Operation mode, index polarity", "type"=enum."U16", "rw"=enum."rw", "lowLimit"="0", "highLimit"="0x9F07", "Default"="0x0", "Kommentart"=""}, {"ID"=588578818, "Name"="Motor encoder_IE resolution", "type"=enum."U32", "rw"=enum."rw", "lowLimit"="0", "highLimit"="4194304", "Default"="", "Kommentart"=""}, {"ID"=588578819, "Name"="Motor encoder_Motor encoder position", "type"=enum."S32", "rw"=enum."ro", "lowLimit"="", "highLimit"="", "Default"="", "Kommentart"=""}, {"ID"=588578820, "Name"="Motor encoder_Gain  (numerator/divisor)", "type"=enum."S32", "rw"=enum."rw", "lowLimit"="-2147483648", "highLimit"="2147483647", "Default"="0x40004000", "Kommentart"=""}, {"ID"=588578821, "Name"="Motor encoder_MotorEnc scaled position", "type"=enum."S32", "rw"=enum."rw", "lowLimit"="-2147483648", "highLimit"="2147483647", "Default"="", "Kommentart"=""}, {"ID"=588578822, "Name"="Motor encoder_Absolute encoder bits", "type"=enum."U32", "rw"=enum."rw", "lowLimit"="0x0", "highLimit"="4294967295", "Default"="", "Kommentart"=""}, {"ID"=588578823, "Name"="Motor encoder_Encoder status", "type"=enum."U8", "rw"=enum."ro", "lowLimit"="", "highLimit"="", "Default"="0", "Kommentart"=""}, {"ID"=588578824, "Name"="Motor encoder_Motor encoder act speed", "type"=enum."S32", "rw"=enum."ro", "lowLimit"="", "highLimit"="", 
